vi "plot_selector2.vi"(4 "\"0\" drift in":cluster{"1":dbl, "2":dbl, "3":dbl, "4":dbl}, 5 "LegendON":bool, 6 "data lables":string[](array[string]), 7 "selector":T1={"data select"={"data1"=1, "data2"=0, "data3"=0, "data4"=0}, "plot color"={"color1"=1, "color2"=1, "color3"=0, "color4"=0}} {"data select"."data4" items=["–", "17_04_14\\10_24_32ch#1", "17_04_14\\10_24_32ch#2", "17_04_14\\10_24_32ch#3", "17_04_14\\10_24_32ch#4", "17_04_14\\10_24_32ch#5", "17_04_14\\10_24_32ch#6", "17_04_14\\10_24_32ch#7", "17_04_14\\10_24_32ch#8", "17_04_14\\10_24_32ch#9", "17_04_14\\10_24_32ch#10", "17_04_14\\10_24_32ch#11", "17_04_14\\10_24_32ch#12", "17_04_14\\10_24_32ch#13", "17_04_14\\10_24_32ch#14", "17_04_14\\10_24_32ch#15", "17_04_14\\10_24_32ch#16", "17_04_14\\10_24_32ch#17", "17_04_14\\10_24_32ch#18", "17_04_14\\10_24_32ch#19", "17_04_14\\10_24_32ch#20", "17_04_14\\10_24_32ch#21", "17_04_14\\10_24_32ch#22", "17_04_14\\10_24_32ch#23", "17_04_14\\10_24_32ch#24", "17_04_14\\10_24_32ch#25", "17_04_14\\10_24_32ch#26", "17_04_14\\10_24_32ch#27", "17_04_14\\10_24_32ch#28", "17_04_14\\10_24_32ch#29", "17_04_14\\10_24_32ch#30"]; "data select"."data3" items=["–", "17_04_14\\10_24_32ch#1", "17_04_14\\10_24_32ch#2", "17_04_14\\10_24_32ch#3", "17_04_14\\10_24_32ch#4", "17_04_14\\10_24_32ch#5", "17_04_14\\10_24_32ch#6", "17_04_14\\10_24_32ch#7", "17_04_14\\10_24_32ch#8", "17_04_14\\10_24_32ch#9", "17_04_14\\10_24_32ch#10", "17_04_14\\10_24_32ch#11", "17_04_14\\10_24_32ch#12", "17_04_14\\10_24_32ch#13", "17_04_14\\10_24_32ch#14", "17_04_14\\10_24_32ch#15", "17_04_14\\10_24_32ch#16", "17_04_14\\10_24_32ch#17", "17_04_14\\10_24_32ch#18", "17_04_14\\10_24_32ch#19", "17_04_14\\10_24_32ch#20", "17_04_14\\10_24_32ch#21", "17_04_14\\10_24_32ch#22", "17_04_14\\10_24_32ch#23", "17_04_14\\10_24_32ch#24", "17_04_14\\10_24_32ch#25", "17_04_14\\10_24_32ch#26", "17_04_14\\10_24_32ch#27", "17_04_14\\10_24_32ch#28", "17_04_14\\10_24_32ch#29", "17_04_14\\10_24_32ch#30"]; "data select"."data2" items=["–", "17_04_14\\10_24_32ch#1", "17_04_14\\10_24_32ch#2", "17_04_14\\10_24_32ch#3", "17_04_14\\10_24_32ch#4", "17_04_14\\10_24_32ch#5", "17_04_14\\10_24_32ch#6", "17_04_14\\10_24_32ch#7", "17_04_14\\10_24_32ch#8", "17_04_14\\10_24_32ch#9", "17_04_14\\10_24_32ch#10", "17_04_14\\10_24_32ch#11", "17_04_14\\10_24_32ch#12", "17_04_14\\10_24_32ch#13", "17_04_14\\10_24_32ch#14", "17_04_14\\10_24_32ch#15", "17_04_14\\10_24_32ch#16", "17_04_14\\10_24_32ch#17", "17_04_14\\10_24_32ch#18", "17_04_14\\10_24_32ch#19", "17_04_14\\10_24_32ch#20", "17_04_14\\10_24_32ch#21", "17_04_14\\10_24_32ch#22", "17_04_14\\10_24_32ch#23", "17_04_14\\10_24_32ch#24", "17_04_14\\10_24_32ch#25", "17_04_14\\10_24_32ch#26", "17_04_14\\10_24_32ch#27", "17_04_14\\10_24_32ch#28", "17_04_14\\10_24_32ch#29", "17_04_14\\10_24_32ch#30"]; "data select"."data1" items=["–", "17_04_14\\10_24_32ch#1", "17_04_14\\10_24_32ch#2", "17_04_14\\10_24_32ch#3", "17_04_14\\10_24_32ch#4", "17_04_14\\10_24_32ch#5", "17_04_14\\10_24_32ch#6", "17_04_14\\10_24_32ch#7", "17_04_14\\10_24_32ch#8", "17_04_14\\10_24_32ch#9", "17_04_14\\10_24_32ch#10", "17_04_14\\10_24_32ch#11", "17_04_14\\10_24_32ch#12", "17_04_14\\10_24_32ch#13", "17_04_14\\10_24_32ch#14", "17_04_14\\10_24_32ch#15", "17_04_14\\10_24_32ch#16", "17_04_14\\10_24_32ch#17", "17_04_14\\10_24_32ch#18", "17_04_14\\10_24_32ch#19", "17_04_14\\10_24_32ch#20", "17_04_14\\10_24_32ch#21", "17_04_14\\10_24_32ch#22", "17_04_14\\10_24_32ch#23", "17_04_14\\10_24_32ch#24", "17_04_14\\10_24_32ch#25", "17_04_14\\10_24_32ch#26", "17_04_14\\10_24_32ch#27", "17_04_14\\10_24_32ch#28", "17_04_14\\10_24_32ch#29", "17_04_14\\10_24_32ch#30"]}, 8 "cut data":refnum<vi>) -> (2 "\"0\" drift out":dbl[](array[numeric]), 3 "data #":i32[](array[numeric]))   [LabVIEW 2014]
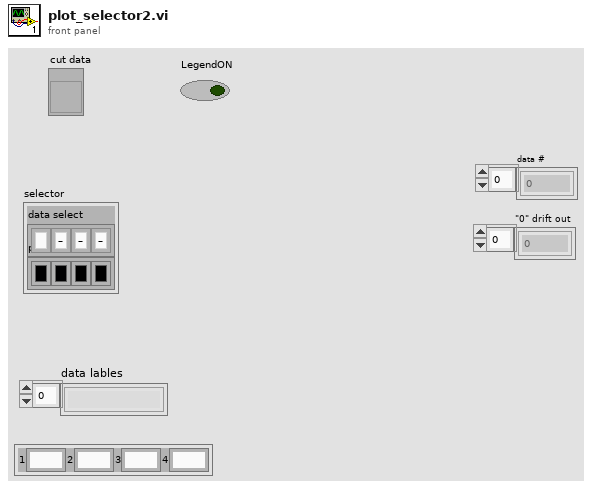
[diagram p1: front panel]
types:
  T1 = cluster{"data select":cluster{"data1":u16, "data2":u16, "data3":u16, "data4":u16}, "plot color":cluster{"color1":u32, "color2":u32, "color3":u32, "color4":u32}}
  T2 = cluster{"color1":u32, "color2":u32, "color3":u32, "color4":u32}
  T3 = cluster{"data1":u16, "data2":u16, "data3":u16, "data4":u16}
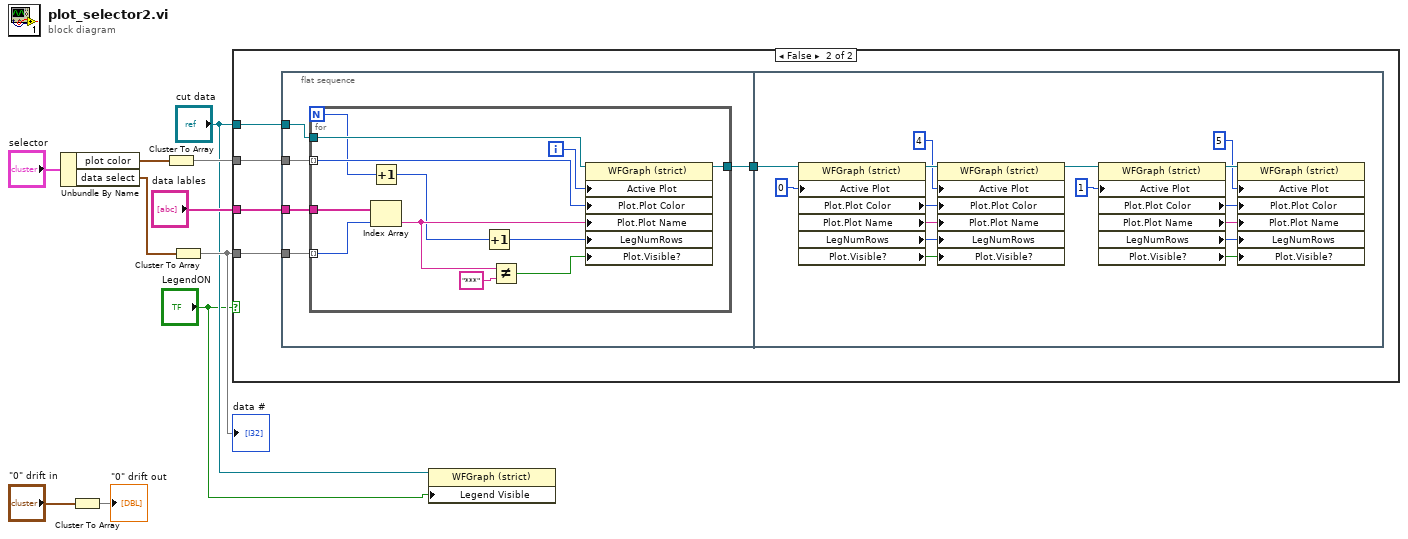
[diagram p0: block diagram]
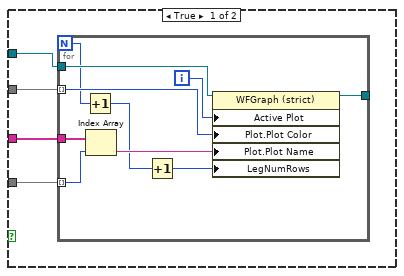
[diagram p2: hidden frame]
diagram:
  n1 = Unbundle By Name("selector") -> ("plot color"=w6:T2, "data select"=w7:T3)
  n2 = Cluster To Array(cluster="\"0\" drift in") -> (array=→"\"0\" drift out":dbl[])
  n3 = Cluster To Array(cluster=w6) -> (array=w5:u32[])
  n4 = Cluster To Array(cluster=w7) -> (array=w4:u16[])
  "data #" <- w4
  n5 = case shown="False" "LegendON" {
    tunnel: w5 -> [w14 w28]
    tunnel: w4 -> [w13 w27]
    tunnel: "cut data" -> [w12 w26]
    tunnel: "data lables" -> [w11 w25]
    frame True {
      n6 = for {
        N -> [w18]
        tunnel: w12 -> [w24]
        tunnel: w13 -> [w20] mode=indexing
        tunnel: w14 -> [w23] mode=indexing
        tunnel: w11 -> [w21]
        tunnel: [w15] -> _
        i -> [w22]
        n7 = Increment(x=w18) -> (x+1=w17:i32)
        n8 = Index Array(array=w21, index=w20) -> (element=w19:string)
        n9 = Increment(x=w17) -> (x+1=w16:i32)
        n10 = property on="Property Node" class="WFGraph (strict)"(reference=w24, "Active Plot"=w22, "Plot.Plot Color"=w23, "Plot.Plot Name"=w19, "LegNumRows"=w16) -> (reference out=w15:refnum<vi>)  [unwired: 1 in, 1 out]
      }
    }
    frame False {
      n11 = flat-sequence {
        tunnel: [w30] -> w29
        tunnel: w28 -> [w34]
        tunnel: w27 -> [w33]
        tunnel: w26 -> [w32]
        tunnel: w25 -> [w31]
        tunnel: w29 -> [w57]
        frame #0 {
          n12 = for {
            N -> [w39]
            tunnel: w32 -> [w46]
            tunnel: w33 -> [w42] mode=indexing
            tunnel: w34 -> [w45] mode=indexing
            tunnel: w31 -> [w43]
            tunnel: [w35] -> w30
            i -> [w44]
            n13 = Increment(x=w39) -> (x+1=w38:i32)
            n14 = Index Array(array=w43, index=w42) -> (element=w41:string)
            n15 = Increment(x=w38) -> (x+1=w37:i32)
            n16 = Not Equal?(x=w41, y="***") -> (x != y?=w36:bool)
            n17 = property on="Property Node" class="WFGraph (strict)"(reference=w46, "Active Plot"=w44, "Plot.Plot Color"=w45, "Plot.Plot Name"=w41, "LegNumRows"=w37, "Plot.Visible?"=w36) -> (reference out=w35:refnum<vi>)  [unwired: 1 in, 1 out]
          }
        }
        frame #1 {
          n18 = property on="Property Node" class="WFGraph (strict)"(reference=w57, "Active Plot"=u32 0) -> (reference out=w50:refnum<vi>, "Plot.Plot Color"=w59:u32, "Plot.Plot Name"=w60:string, "LegNumRows"=w61:u32, "Plot.Visible?"=w62:bool)  [unwired: 1 in, 1 out]
          n19 = property on="Property Node" class="WFGraph (strict)"(reference=w50, "Active Plot"=u32 4, "Plot.Plot Color"=w59, "Plot.Plot Name"=w60, "LegNumRows"=w61, "Plot.Visible?"=w62) -> (reference out=w51:refnum<vi>)  [unwired: 1 in, 1 out]
          n20 = property on="Property Node" class="WFGraph (strict)"(reference=w51, "Active Plot"=u32 1) -> (reference out=w49:refnum<vi>, "Plot.Plot Color"=w53:u32, "Plot.Plot Name"=w54:string, "LegNumRows"=w55:u32, "Plot.Visible?"=w56:bool)  [unwired: 1 in, 1 out]
          n21 = property on="Property Node" class="WFGraph (strict)"(reference=w49, "Active Plot"=u32 5, "Plot.Plot Color"=w53, "Plot.Plot Name"=w54, "LegNumRows"=w55, "Plot.Visible?"=w56) -> ()  [unwired: 1 in, 2 out]
        }
      }
    }
  }
  n22 = property class="WFGraph (strict)"(reference="cut data", "Legend Visible"="LegendON") -> ()  [unwired: 1 in, 2 out]
